vi "reset.vi"(0 "Interface in":T1, 11 "error in":errorcluster) -> (4 "Interface out":T1, 15 "error out":errorcluster)   [LabVIEW 2017, in "ThreePhasePLLInterface.lvlib"]
uses:
  ThreePhasePLLInterface.lvlib
  InterfaceRef.ctl
  <instrlib>/_niInstr/Instruction Framework/v1/Host/Instruction Target/niInstr Instruction Target v1 Host.lvclass
  <instrlib>/_niInstr/Instruction Framework/v1/Host/Instruction Framework Context/niInstr Instruction Framework Context v1 Host.lvclass
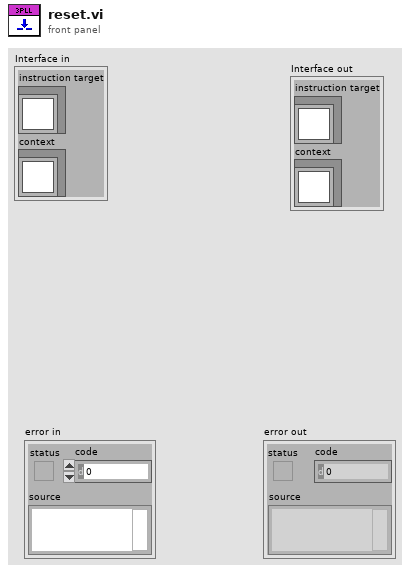
[diagram p1: front panel]
types:
  T1 = typedef "ThreePhasePLLInterface.lvlib/InterfaceRef.ctl" = cluster{"instruction target":refnum<class "niInstr Instruction Target v1 Host.lvclass">, "context":refnum<class "niInstr Instruction Framework Context v1 Host.lvclass">}
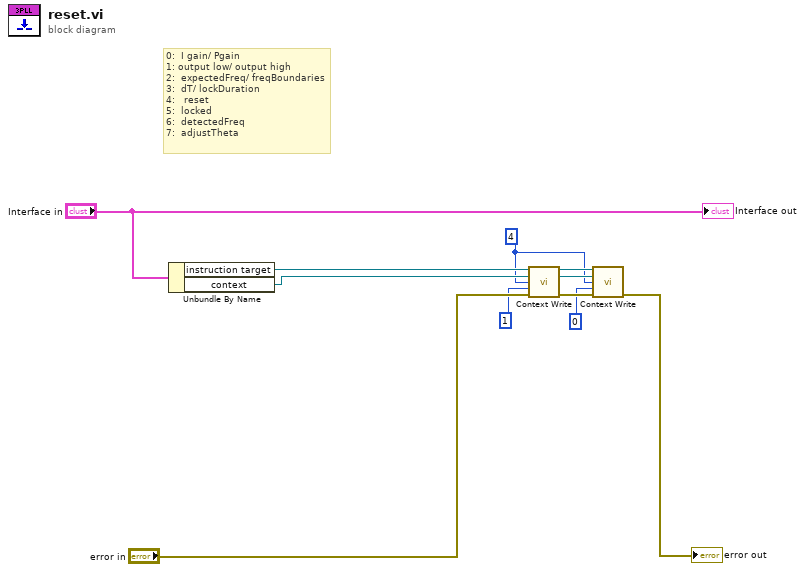
[diagram p0: block diagram]
diagram:
  w3 = u64 4 ("address")
  # "0:  I gain/ Pgain\n1: output low/ output high\n2:  expectedFreq/ freqBoundaries\n3:  dT/ lockDuration\n4:   reset\n5:  locked\n6:  detectedFreq\n7:  adjustTheta"
  n1 = Unbundle By Name("Interface in") -> ("instruction target"=w11:refnum<class "niInstr Instruction Target v1 Host.lvclass">, "context"=w10:refnum<class "niInstr Instruction Framework Context v1 Host.lvclass">)
  n2 = call <instrlib>:"Context Write.vi"("instruction target in"=w11, "context in"=w10, "address"=w3, "data"=u64 1, "error in"="error in") -> ("instruction target out"=w6:refnum<class "niInstr Instruction Target v1 Host.lvclass">, "context out"=w4:refnum<class "niInstr Instruction Framework Context v1 Host.lvclass">, "error out"=w5:errorcluster)  [unwired: 8 in]
  n3 = call <instrlib>:"Context Write.vi"("instruction target in"=w6, "context in"=w4, "address"=w3, "data"=u64 0, "error in"=w5) -> ("error out"=→"error out":errorcluster)  [unwired: 8 in, 2 out]
  "Interface out" <- "Interface in"
